vi "Window_MeassurementName.vi"() -> ()   [LabVIEW 2019]
uses:
  #Praca/Extensa/UserApp GIT/03_Software/#typedefs/#control_StopButton.ctl
  <vilib>/Utility/miscctls.llb/LVRectTypeDef.ctl
  <vilib>/Utility/miscctls.llb/LVPoint32TypeDef.ctl
panel:
  out "Coords":T1
  out "Window Bounds":T2
  out "Is Window Dragged?":bool
  in  "Tab":enum32{"Page 1"}(tab)
  out "WindowHandler":bool=TRUE
  in  "STOP":T3
  out "Komunikat":string caption="Wpisz kod"
  out "error out":errorcluster
  in  "error in (no error)":errorcluster
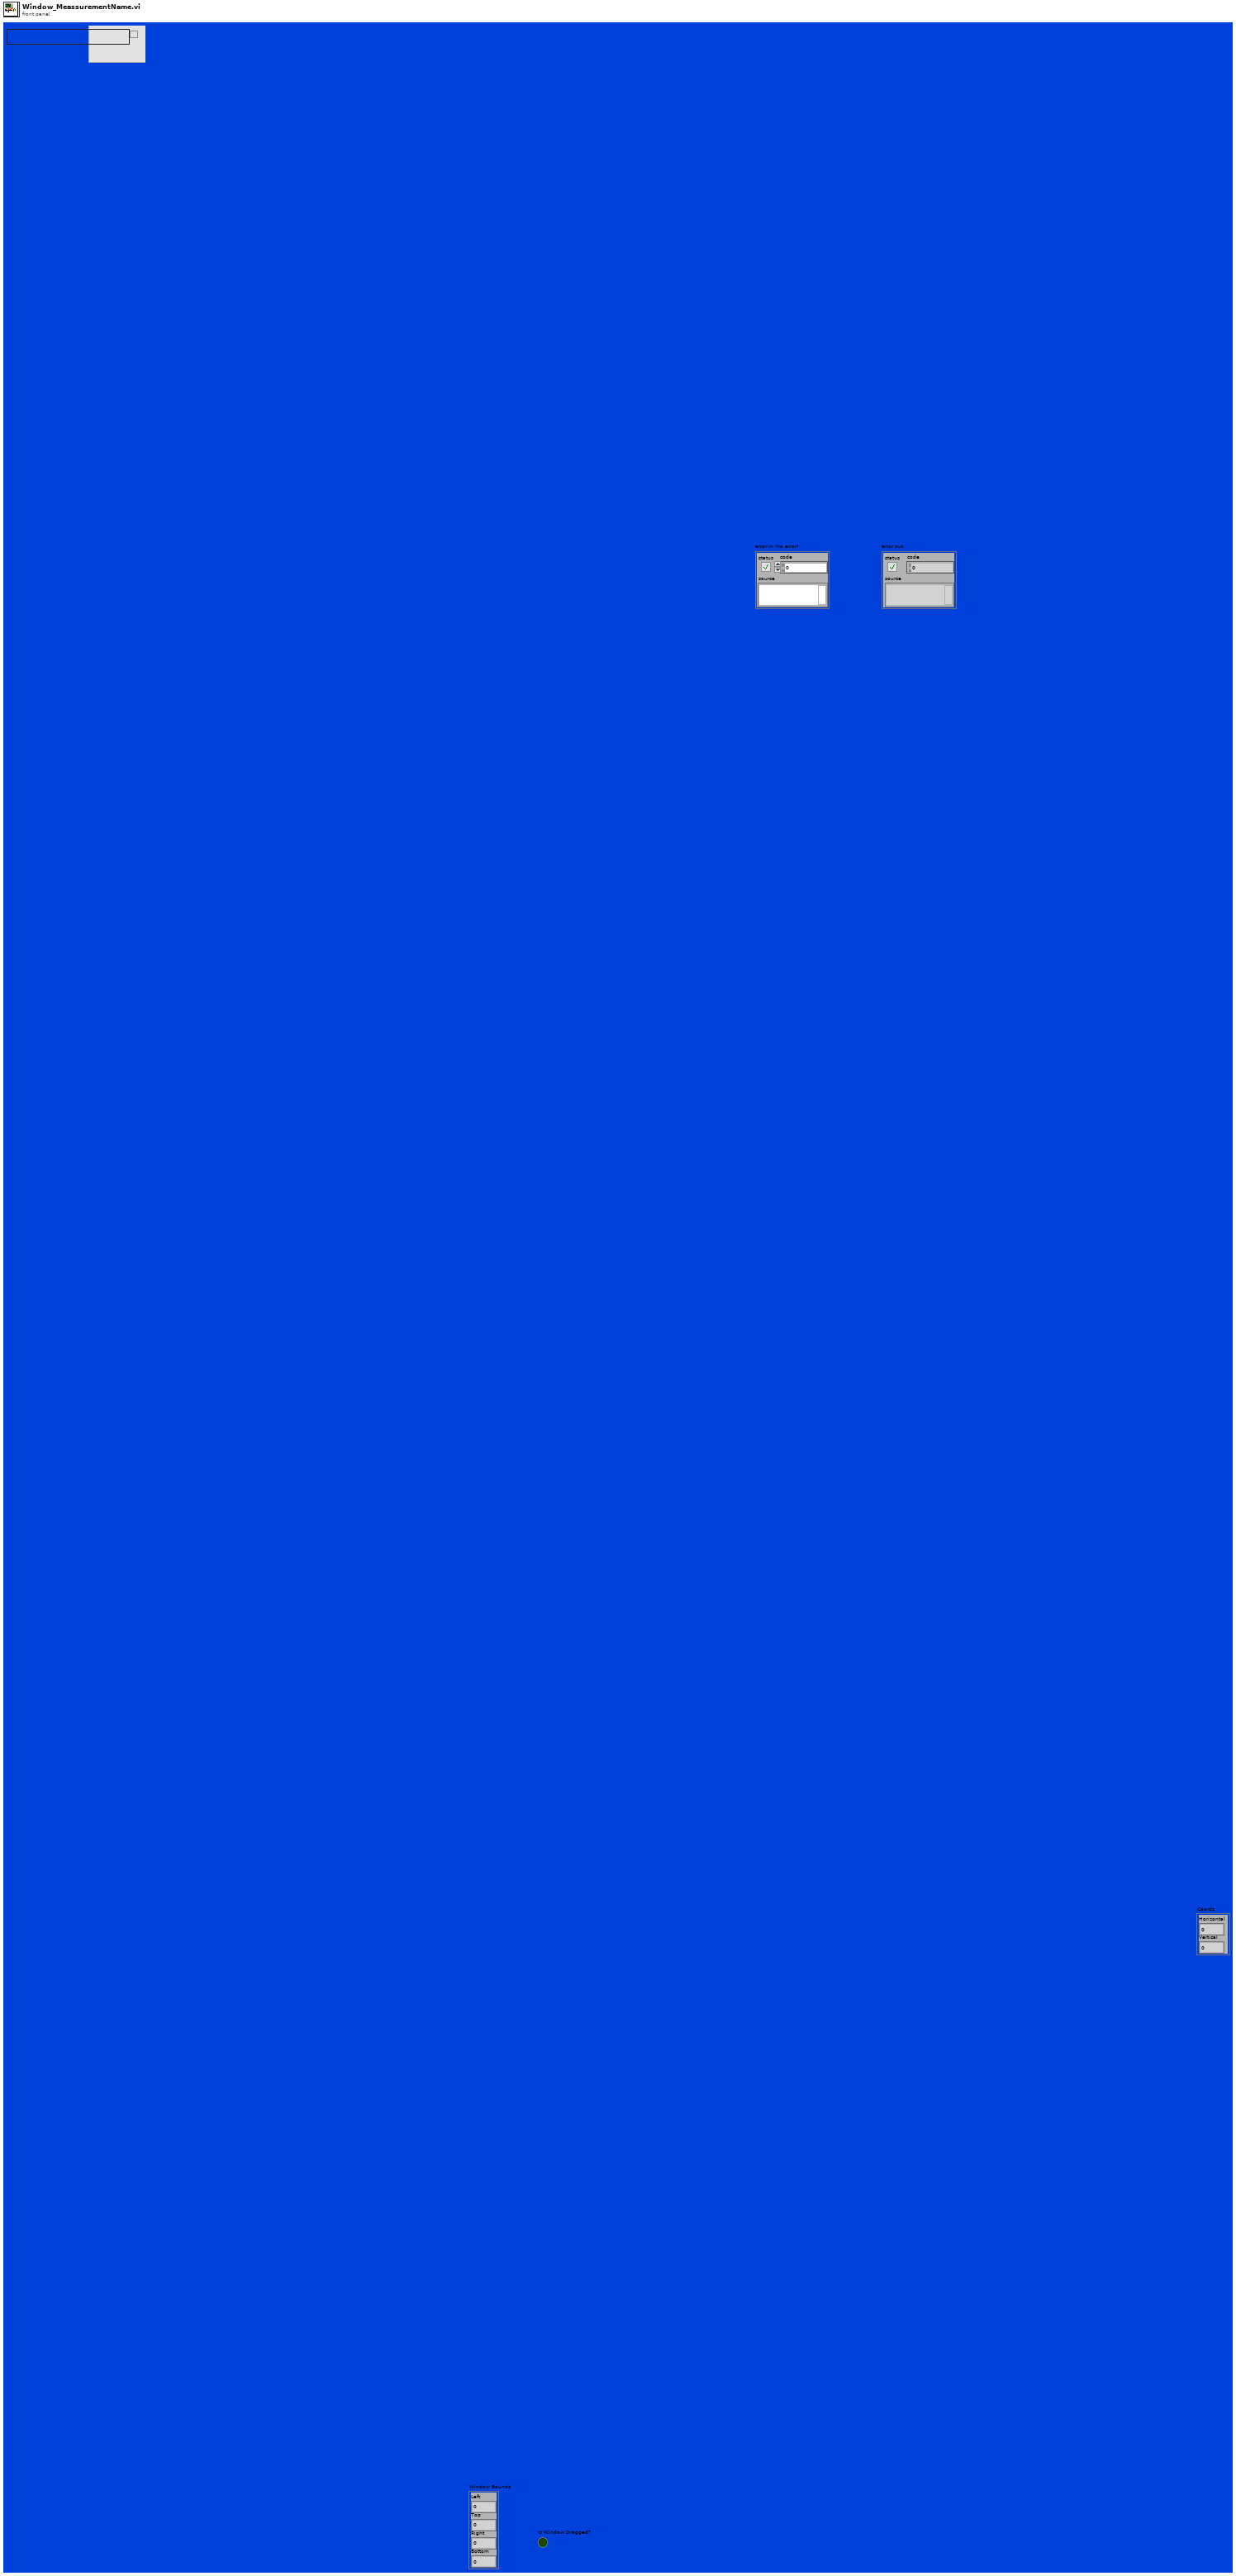
[diagram p1: front panel]
types:
  T1 = typedef "LVPoint32TypeDef.ctl" = cluster{"Horizontal":i32, "Vertical":i32}
  T2 = typedef "LVRectTypeDef.ctl" = cluster{"Left":i16, "Top":i16, "Right":i16, "Bottom":i16}
  T3 = typedef "#control_StopButton.ctl" = bool
  T4 = cluster{"Horizontal":i16, "Vertical":i16, "Horizontal":i16, "Vertical":i16}
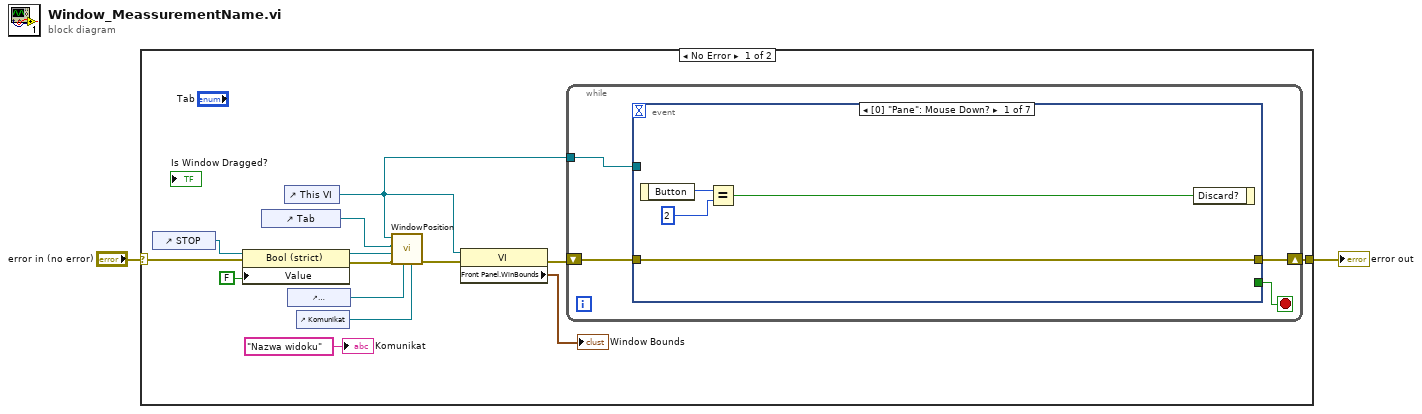
[diagram p0: block diagram]
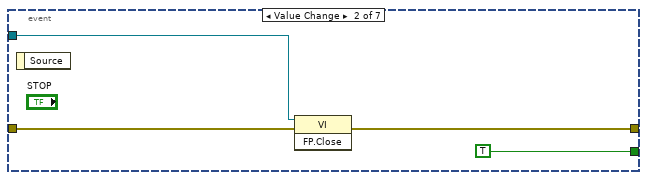
[diagram p2: hidden frame]
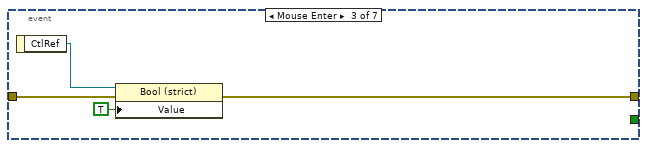
[diagram p3: hidden frame]
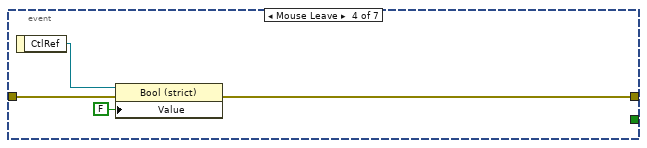
[diagram p4: hidden frame]
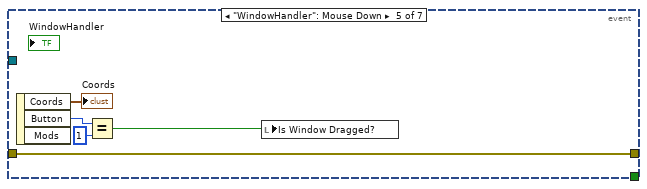
[diagram p5: hidden frame]
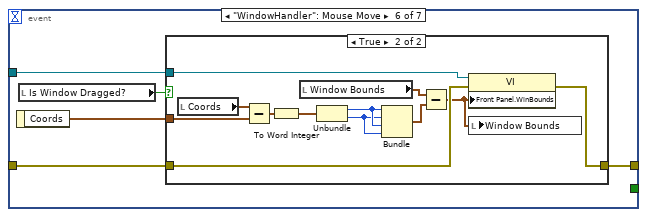
[diagram p6: hidden frame]
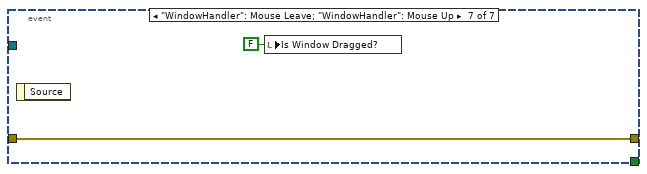
[diagram p8: hidden frame]
diagram:
  n1 = case shown="No Error" "error in (no error)" {
    selector: "error in (no error)" -> [w11 w62]
    tunnel: [w16 w62] -> w2
    frame No Error {
      n2 = control-ref of="STOP"() -> (w12:refnum<vi>)
      n3 = property class="Bool (strict)"(reference=w12, error in=w11, "Value"=T3 FALSE) -> (reference out=w4:refnum<vi>, error out=w8:errorcluster)
      n4 = control-ref of="Tab"() -> (w6:refnum<vi>)
      n5 = control-ref of="This VI"() -> (w5:refnum<vi>)
      n6 = control-ref of="WindowHandler"() -> (w3:refnum<vi>)
      n7 = control-ref of="Komunikat"() -> (w7:refnum<vi>)
      n8 = call "WindowPosition.vi"("Komunikat"=w7, "WindowHandler"=w3, "error in (no error)"=w8, "STOP"=w4, "Tab"=w6, "VI in"=w5) -> ("error out"=w9:errorcluster)  [unwired: 5 in]
      n9 = property class="VI"(reference=w5, error in=w9) -> (error out=w15:errorcluster, "Front Panel.WinBounds"=→"Window Bounds":T2)  [unwired: 1 out]
      n10 = while {
        shift-right: [w18] -> w16
        shift-left: w15 -> [w20]
        tunnel: w5 -> [w17]
        stop <- w19 stop-if-true
        n11 = event shown="[0] \"Pane\": Mouse Down?" {
          selector: _ -> [_ _ _ _ _ _ _]
          dyn-events: _ -> [_ _ _ _ _ _ _]
          timeout: _ -> [_ _ _ _ _ _ _]
          tunnel: w20 -> [w21 w28 w31 w35 w37 w44 w60]
          tunnel: [w21 w27 w30 w34 w37 w43 w60] -> w18
          tunnel: [_ TRUE _ _ _ _ _] -> w19
          tunnel: w17 -> [_ w25 _ _ _ w42 _]
          event Mouse Down? {
            n12 = event-data() -> ("Button"=w24:u16)  [unwired: 1 in]
            n13 = Equal?(x=w24, y=u16 2) -> (x = y?=w22:bool)
            n14 = event-data("Discard?"=w22) -> ()  [unwired: 1 in, 1 out]
          }
          event Value Change {
            n15 = event-data() -> ()  [unwired: 1 in, 1 out]
            n16 = invoke class="VI" method="FP.Close"(reference=w25, error in=w28) -> (error out=w27:errorcluster)  [unwired: 1 in, 2 out]
          }
          event Mouse Enter {
            n17 = event-data() -> ("CtlRef"=w32:refnum<vi>)  [unwired: 1 in]
            n18 = property class="Bool (strict)"(reference=w32, error in=w31, "Value"=T3 TRUE) -> (error out=w30:errorcluster)  [unwired: 1 out]
          }
          event Mouse Leave {
            n19 = event-data() -> ("CtlRef"=w36:refnum<vi>)  [unwired: 1 in]
            n20 = property class="Bool (strict)"(reference=w36, error in=w35, "Value"=T3 FALSE) -> (error out=w34:errorcluster)  [unwired: 1 out]
          }
          event "WindowHandler": Mouse Down {
            n21 = event-data() -> ("Coords"=→"Coords":T1, "Button"=w40:u16)  [unwired: 1 in, 1 out]
            n22 = Equal?(x=w40, y=u16 1) -> (x = y?=w38:bool)
            n23 = local write "Is Window Dragged?"(w38) -> ()
          }
          event "WindowHandler": Mouse Move {
            n24 = event-data() -> ("Coords"=w45:T1)  [unwired: 1 in]
            n25 = local read "Is Window Dragged?"() -> (w46:bool)
            n26 = case shown="True" w46 {
              tunnel: w45 -> [_ w54]
              tunnel: w44 -> [w47 w51]
              tunnel: [w47 w50] -> w43
              tunnel: w42 -> [_ w48]
              frame False {
              }
              frame True {
                n27 = local read "Coords"() -> (w55:T1)
                n28 = Subtract(x=w55, y=w54) -> (x-y=w59:T1)
                n29 = To Word Integer(number=w59) -> (16bit integer=w58:cluster{"Horizontal":i16, "Vertical":i16})
                n30 = local read "Window Bounds"() -> (w53:T2)
                n31 = Unbundle(w58) -> ("Horizontal"=w57:i16, "Vertical"=w56:i16)
                n32 = Bundle("Horizontal"=w57, "Vertical"=w56, "Horizontal"=w57, "Vertical"=w56) -> (w52:T4)  [unwired: 1 in]
                n33 = Subtract(x=w53, y=w52) -> (x-y=w49:T2)
                n34 = property class="VI"(reference=w48, error in=w51, "Front Panel.WinBounds"=w49) -> (error out=w50:errorcluster)  [unwired: 1 out]
                n35 = local write "Window Bounds"(w49) -> ()
              }
            }
          }
          event "WindowHandler": Mouse Leave; "WindowHandler": Mouse Up {
            n36 = event-data() -> ()  [unwired: 1 in, 1 out]
            n37 = local write "Is Window Dragged?"(FALSE ("Is Window Dragged?")) -> ()
          }
        }
      }
      "Komunikat" <- "Nazwa widoku" ("Komunikat")
    }
    frame Error {
    }
  }
  "error out" <- w2
